vi "FTW-Listener-Wait On Connection.vi"(0 "FTW-Listener-LVQ In":refnum<class "FTW-Listener-LVQ.lvclass">, 11 "error in":errorcluster) -> (4 "FTW-Listener-LVQ Out":refnum<class "FTW-Listener-LVQ.lvclass">, 6 "Endpoint":refnum<class "FTW-Endpoint.lvclass">, 15 "error out":errorcluster)   [LabVIEW 2013, in "FTW-Listener-LVQ.lvclass"]
uses:
  FTW-Listener-LVQ.lvclass
  Endpoint/FTW-Endpoint.lvclass
  FTW-Listener-LVQ.lvclass/FTW-Listener-LVQ.ctl
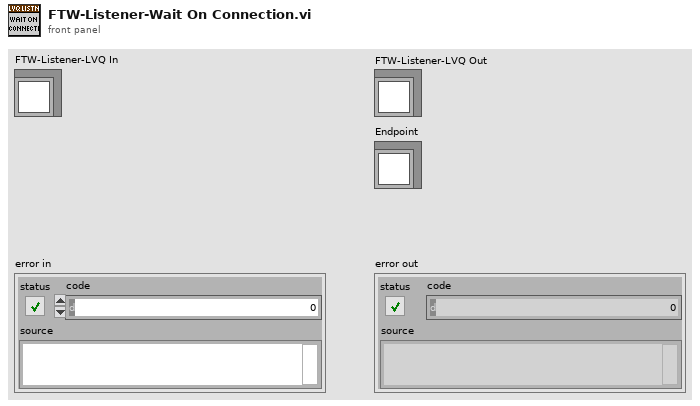
[diagram p1: front panel]
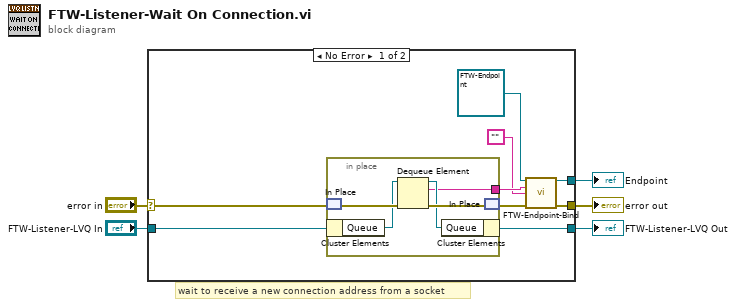
[diagram p0: block diagram]
diagram:
  # "wait to receive a new connection address from a socket"
  n1 = case shown="No Error" "error in" {
    selector: "error in" -> [w13 w21]
    tunnel: [w10 w21] -> w4
    tunnel: [w14 w20] -> w3
    tunnel: "FTW-Listener-LVQ In" -> [w12 w20]
    tunnel: [w9 _] -> w1
    frame No Error {
      n2 = in-place {
        in-place-border: [w15] -> w8
        n3 = in-place-match #1(w13) -> (w19:errorcluster)
        n4 = in-place-cluster #2(w12) -> ("Queue"=w18:refnum<queue>)
        n5 = Dequeue Element(queue=w18, error in (no error)=w19) -> (queue out=w16:refnum<queue>, element=w15:string, error out=w17:errorcluster)  [unwired: 1 in, 1 out]
        n6 = in-place-cluster #2("Queue"=w16) -> (w14:refnum<class "FTW-Listener-LVQ.lvclass">)
        n7 = in-place-match #1(w17) -> (w11:errorcluster)
      }
      n8 = call-dynamic "FTW-Endpoint-Bind.vi"("FTW Endpoint"=refnum<class "FTW-Endpoint.lvclass"> refnum, "Endpoint Address"=w8, "Requested Identity"="", "error in"=w11) -> ("FTW Endpoint out"=w9:refnum<class "FTW-Endpoint.lvclass">, "error out"=w10:errorcluster)  [unwired: 8 in, 2 out]
    }
    frame Error {
    }
  }
  "FTW-Listener-LVQ Out" <- w3
  "error out" <- w4
  "Endpoint" <- w1
